vi "Convert_RGB_to_Irradience.vi"(8 "Unfiltered":u16, 9 "B":u16, 10 "G":u16, 11 "R":u16) -> (0 "Unfiltered":dbl, 1 "B":dbl, 2 "G":dbl, 3 "R":dbl)   [LabVIEW 2018]
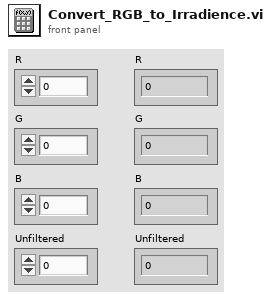
[diagram p1: front panel]
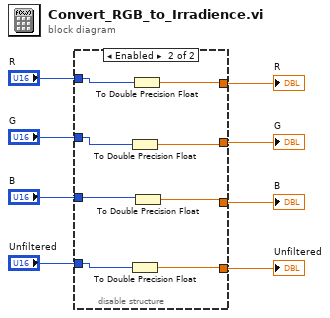
[diagram p0: block diagram]
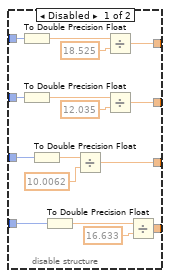
[diagram p2: hidden frame]
diagram:
  n1 = disable-structure shown="Enabled" {
    disable-tunnel: "Unfiltered" -> [w20 w26]
    disable-tunnel: "B" -> [w19 w28]
    disable-tunnel: "G" -> [w18 w30]
    disable-tunnel: "R" -> [w17 w32]
    disable-tunnel: [w16 w31] -> w4
    disable-tunnel: [w15 w29] -> w3
    disable-tunnel: [w14 w27] -> w2
    disable-tunnel: [w13 w25] -> w1
    frame Disabled {
      n2 = To Double Precision Float(number=w17) -> (double precision float=w12:dbl)
      n3 = To Double Precision Float(number=w18) -> (double precision float=w11:dbl)
      n4 = To Double Precision Float(number=w19) -> (double precision float=w10:dbl)
      n5 = To Double Precision Float(number=w20) -> (double precision float=w9:dbl)
      n6 = Divide(x=w10, y=10.0062 ("x")) -> (x/y=w14:dbl)
      n7 = Divide(x=w12, y=18.525 ("x")) -> (x/y=w16:dbl)
      n8 = Divide(x=w11, y=12.035 ("x")) -> (x/y=w15:dbl)
      n9 = Divide(x=w9, y=16.633 ("x")) -> (x/y=w13:dbl)
    }
    frame Enabled {
      n10 = To Double Precision Float(number=w30) -> (double precision float=w29:dbl)
      n11 = To Double Precision Float(number=w26) -> (double precision float=w25:dbl)
      n12 = To Double Precision Float(number=w32) -> (double precision float=w31:dbl)
      n13 = To Double Precision Float(number=w28) -> (double precision float=w27:dbl)
    }
  }
  "R" <- w4
  "G" <- w3
  "B" <- w2
  "Unfiltered" <- w1
